vi "globalSetUp.vi"(8 "error in (no error)":errorcluster, 11 "testcase-CSMNonCSMCallerSupportAPI.lvclass in":refnum<class "testcase-CSMNonCSMCallerSupportAPI.lvclass">) -> (0 "error out":errorcluster, 3 "testcase-CSMNonCSMCallerSupportAPI.lvclass out":refnum<class "testcase-CSMNonCSMCallerSupportAPI.lvclass">)   [LabVIEW 2017, in "testcase-CSMNonCSMCallerSupportAPI.lvclass"]
uses:
  testcase-CSMNonCSMCallerSupportAPI.lvclass
  <vilib>/addons/_JKI Toolkits/VI Tester/TestCase.llb/TestCase.lvclass
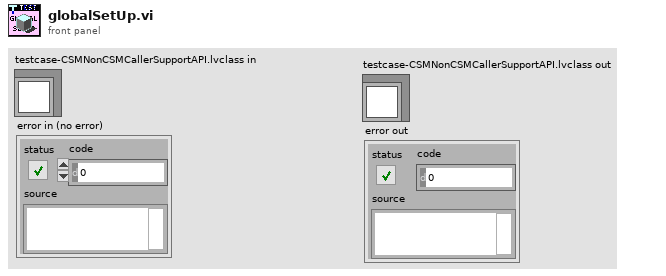
[diagram p1: front panel]
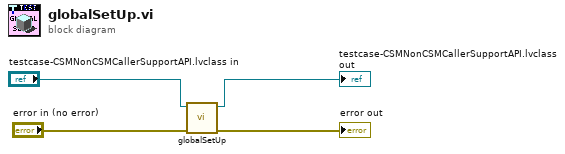
[diagram p0: block diagram]
diagram:
  n1 = call-parent "globalSetUp.vi"("error in (no error)"="error in (no error)", "TestCase in"="testcase-CSMNonCSMCallerSupportAPI.lvclass in") -> ("error out"=→"error out":errorcluster, "TestCase out"=→"testcase-CSMNonCSMCallerSupportAPI.lvclass out":refnum<class "testcase-CSMNonCSMCallerSupportAPI.lvclass">)  [unwired: 8 in]
